vi "pulse-laser_2017.10.25.vi"() -> ()   [LabVIEW 2014]
panel:
  in  "exit":bool
  in  "start":bool
  in  "frequency_Hz":dbl format="%#_6p"
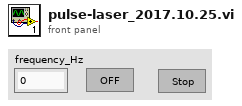
[diagram p1: front panel]
types:
  T1 = cluster{"Instruct Data":i32, "Op Code":i32, "Flags":bool[], "Comments":string, "Time":dbl}
  T2 = cluster{"Instruct Data":i32, "Op Code":i32, "Flags":bool[], "Comments":string, "Time":dbl}[]
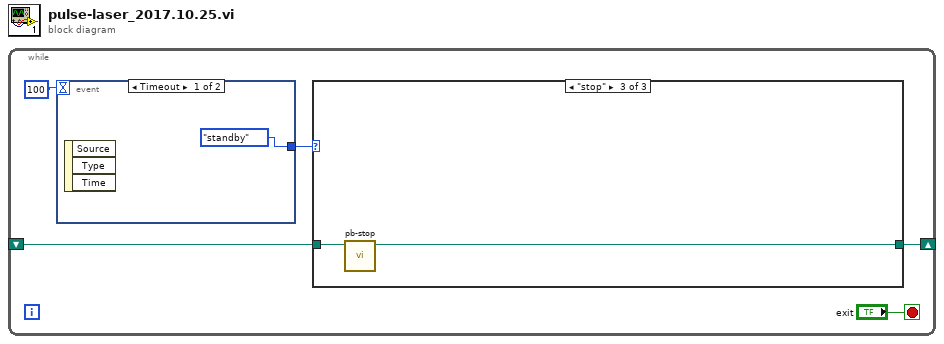
[diagram p0: block diagram]
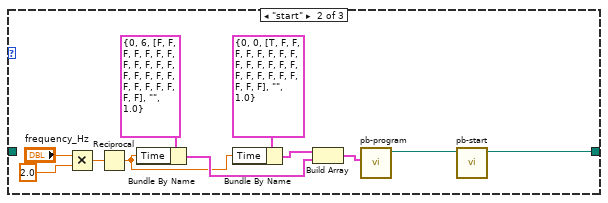
[diagram p3: hidden frame]
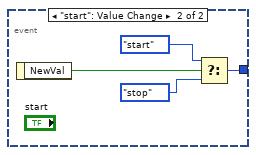
[diagram p4: hidden frame]
diagram:
  n1 = while {
    shift-right: [w4] -> _
    shift-left: _ -> [w3]
    stop <- "exit" stop-if-true
    n2 = event shown="[0] Timeout" {
      selector: _ -> [_ _]
      dyn-events: _ -> [_ _]
      timeout: 100 -> [_ _]
      tunnel: [enum16{"standby", "start", "stop"}."standby" w24] -> w2
      event Timeout {
        n3 = event-data() -> ()  [unwired: 1 in, 3 out]
      }
      event "start": Value Change {
        n4 = event-data() -> ("NewVal"=w22:bool)  [unwired: 1 in]
        n5 = Select(t=enum16{"standby", "start", "stop"}."start", s=w22, f=enum16{"standby", "start", "stop"}."stop") -> (s? t:f=w24:enum16{"standby", "start", "stop"})
      }
    }
    n6 = case shown="\"stop\"" w2 {
      tunnel: [w6 w7 w18] -> w4
      tunnel: w3 -> [w6 _ w19]
      frame "standby", Default {
      }
      frame "start" {
        n7 = Multiply(x="frequency_Hz", y=2.0) -> (x*y=w11:dbl)
        n8 = Reciprocal(x=w11) -> (1/x=w10:dbl)
        n9 = Bundle By Name(cluster=T1 {"Instruct Data"=0, "Op Code"=6, "Flags"=[FALSE, FALSE, FALSE, FALSE, FALSE, FALSE, FALSE, FALSE, FALSE, FALSE, FALSE, FALSE, FALSE, FALSE, FALSE, FALSE, FALSE, FALSE, FALSE, FALSE, FALSE, FALSE, FALSE, FALSE], "Comments"="", "Time"=1.0} ("PB Instruction"), "Time"=w10) -> (w14:T1)
        n10 = Bundle By Name(cluster=T1 {"Instruct Data"=0, "Op Code"=0, "Flags"=[TRUE, FALSE, FALSE, FALSE, FALSE, FALSE, FALSE, FALSE, FALSE, FALSE, FALSE, FALSE, FALSE, FALSE, FALSE, FALSE, FALSE, FALSE, FALSE, FALSE, FALSE, FALSE, FALSE, FALSE], "Comments"="", "Time"=1.0} ("PB Instruction"), "Time"=w10) -> (w15:T1)
        n11 = Build Array(w15, w14) -> (w9:T2)
        n12 = call "pb-program.vi"("Commands"=w9) -> ("path out"=w8:path)  [unwired: 10 in]
        n13 = call "pb-start.vi"("path in"=w8) -> ("path out"=w7:path)  [unwired: 10 in]
      }
      frame "stop" {
        n14 = call "pb-stop.vi"("path in"=w19) -> ("path out"=w18:path)  [unwired: 9 in, 1 out]
      }
    }
  }
